vi "Destroy Broadcast Events.vi"(8 "error in":errorcluster) -> (0 "error out":errorcluster)   [LabVIEW 2024, in "MoneyControl.lvlib"]
doc: "Destroy the broadcast events, even if there is an incoming error.\n\n<b>NOTE</b>: The contents of this VI are automatically generated and modified by the <b>Tools > DQMH Consortium > DQMH</b> utilities. Consider using those utilities instead of making your own modifications to this VI.\n_____\nBased on DQMH Dev Tools: Project Template 7.1.0.1503."
uses:
  MoneyControl.lvlib
panel:
  # "NOTE: The contents of this VI are automatically generated and modified by the Tools > DQMH Consortium > DQMH utilities. Consider using those utilities instead of making your own modifications to this VI."
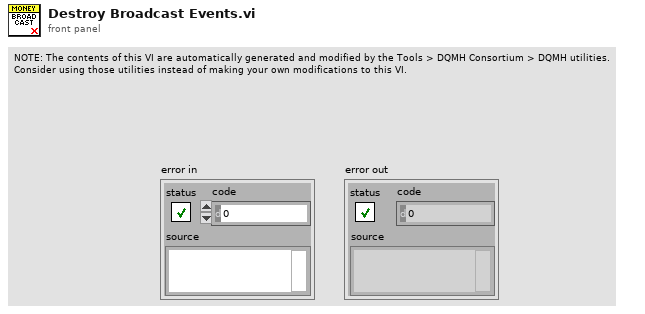
[diagram p1: front panel]
types:
  T1 = typedef "MoneyControl.lvlib/Broadcast Events--cluster.ctl" = cluster{"Module Did Init":refnum<user-event>, "Status Updated":refnum<user-event>, "Error Reported":refnum<user-event>, "Module Did Stop":refnum<user-event>, "Update Module Execution Status":refnum<user-event>, "Credito Actualizado":refnum<user-event>, "Cambio Actualizado":refnum<user-event>}
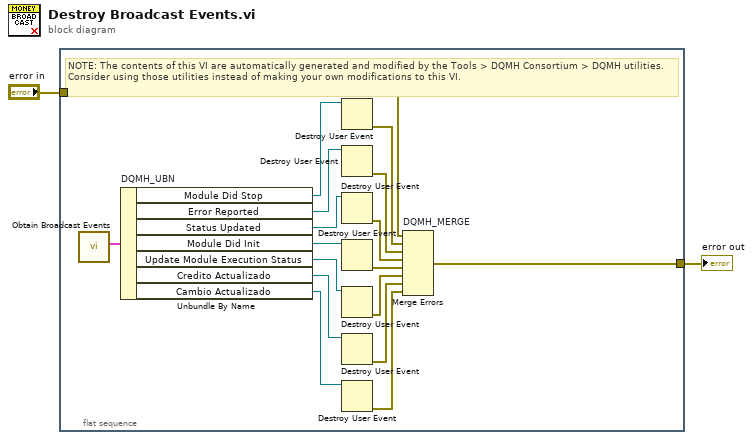
[diagram p0: block diagram]
diagram:
  n1 = flat-sequence {
    tunnel: [w18] -> w2
    tunnel: "error in" -> [w9]
    frame #0 {
      # "NOTE: The contents of this VI are automatically generated and modified by the Tools > DQMH Consortium > DQMH utilities. Consider using those utilities instead of making your own modifications to this VI."
      n2 = call "Obtain Broadcast Events.vi"() -> ("MoneyControl Broadcast Events"=w17:T1)  [unwired: 10 in, 1 out]
      n3 = Unbundle By Name "DQMH_UBN"(w17) -> ("Module Did Stop"=w10:refnum<user-event>, "Error Reported"=w12:refnum<user-event>, "Status Updated"=w15:refnum<user-event>, "Module Did Init"=w16:refnum<user-event>, "Update Module Execution Status"=w7:refnum<user-event>, "Credito Actualizado"=w5:refnum<user-event>, "Cambio Actualizado"=w3:refnum<user-event>)
      n4 = Destroy User Event(user event=w10) -> (error out=w11:errorcluster)  [unwired: 1 in]
      n5 = Destroy User Event(user event=w12) -> (error out=w13:errorcluster)  [unwired: 1 in]
      n6 = Destroy User Event(user event=w15) -> (error out=w14:errorcluster)  [unwired: 1 in]
      n7 = Destroy User Event(user event=w16) -> (error out=w19:errorcluster)  [unwired: 1 in]
      n8 = Destroy User Event(user event=w7) -> (error out=w8:errorcluster)  [unwired: 1 in]
      n9 = Destroy User Event(user event=w5) -> (error out=w6:errorcluster)  [unwired: 1 in]
      n10 = Destroy User Event(user event=w3) -> (error out=w4:errorcluster)  [unwired: 1 in]
      n11 = Merge Errors "DQMH_MERGE"(w9, w11, w13, w14, w19, w8, w6, w4) -> (w18:errorcluster)
    }
  }
  "error out" <- w2
